vi "Write Deadband.vi"(8 "error in (no error)":errorcluster, 10 "Deadband":T1, 11 "Level Controller in":refnum<class "Level Controller.lvclass">) -> (0 "error out":errorcluster, 3 "Level Controller out":refnum<class "Level Controller.lvclass">)   [LabVIEW 2025, in "Level Controller.lvlib" / "Level Controller.lvclass"]
doc: "Writes the deadband range of this Level Controller. The high and low points can be set to the same value, but if the low point is greater than the high point, this method returns error code 1."
uses:
  Level Controller.lvclass
  Deadband.ctl
  Level Controller.lvclass/Level Controller.ctl
  <vilib>/Utility/error.llb/Error Cluster From Error Code.vi
  <vilib>/ErrorRing/Error Ring.xnode
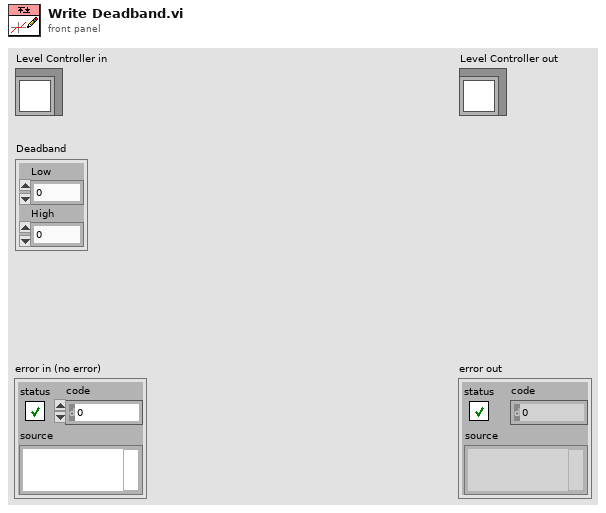
[diagram p1: front panel]
types:
  T1 = typedef "Level Controller.lvlib/Level Controller.lvclass/Deadband.ctl" = cluster{"Low":dbl, "High":dbl}
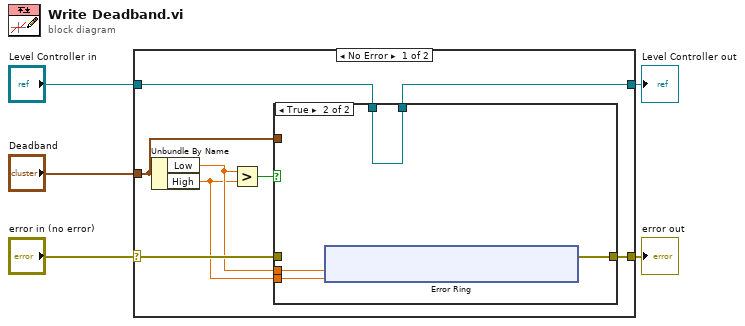
[diagram p0: block diagram]
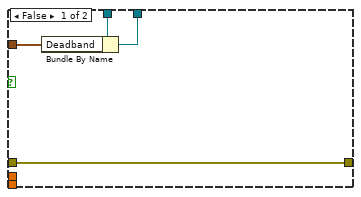
[diagram p2: hidden frame]
diagram:
  n1 = case shown="No Error" "error in (no error)" {
    selector: "error in (no error)" -> [w8 w30]
    tunnel: [w9 w30] -> w4
    tunnel: [w12 w31] -> w2
    tunnel: "Level Controller in" -> [w13 w31]
    tunnel: "Deadband" -> [w10 _]
    frame No Error {
      n2 = Unbundle By Name(w10) -> ("Low"=w7:dbl, "High"=w6:dbl)
      n3 = Greater?(x=w7, y=w6) -> (0:w11:bool)
      n4 = case shown="True" w11 {
        tunnel: w13 -> [w17 w21]
        tunnel: [w16 w21] -> w12
        tunnel: w10 -> [w15 _]
        tunnel: [w14 w20] -> w9
        tunnel: w8 -> [w14 _]
        tunnel: w7 -> [_ w19]
        tunnel: w6 -> [_ w18]
        frame False {
          n5 = Bundle By Name(cluster=w17, "Deadband"=w15) -> (w16:refnum<class "Level Controller.lvclass">)
        }
        frame True {
          n6 = xnode "Error Ring"("parameter 0"=w19, "parameter 1"=w18) -> ("error out"=w20:errorcluster)
        }
      }
    }
    frame Error {
    }
  }
  "error out" <- w4
  "Level Controller out" <- w2
